vi "GC init.vi"(11 "Serial Port":refnum<visa-resource-name>) -> (0 "error":bool, 3 "Serial Port":refnum<visa-resource-name>)   [LabVIEW 2012]
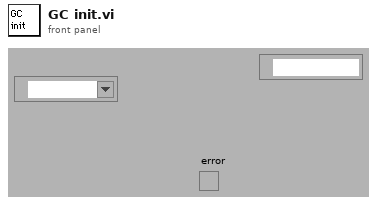
[diagram p1: front panel]
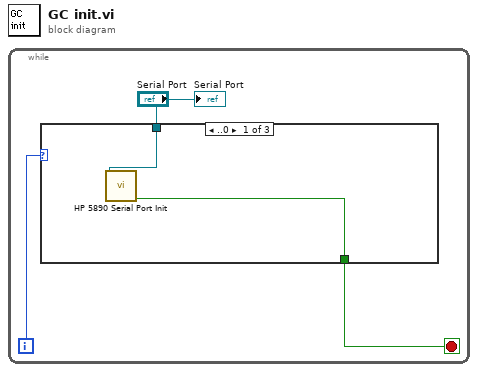
[diagram p0: block diagram]
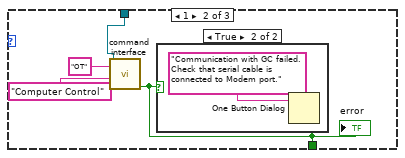
[diagram p2: hidden frame]
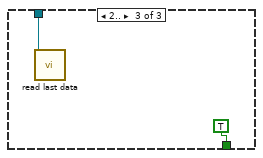
[diagram p4: hidden frame]
diagram:
  n1 = while {
    i -> [w2]
    stop <- w1 stop-if-true
    n2 = case shown="..0" w2 {
      tunnel: "Serial Port" -> [w5 w9 w12]
      tunnel: [w4 w6 TRUE ("timed out")] -> w1
      frame ..0 {
        n3 = call "HP 5890 Serial Port Init.vi"("port number"=w5) -> ("timed out"=w4:bool)  [unwired: 9 in, 1 out]
      }
      frame 1 {
        n4 = call "command interface.vi"("Parameter"="Computer Control", "command"="OT", "Serial Port"=w9) -> ("timed out"=w6:bool)  [unwired: 4 in, 3 out]
        "error" <- w6
        n5 = case shown="True" w6 {
          frame False {
          }
          frame True {
            n6 = One Button Dialog(message="Communication with GC failed. Check that serial cable is connected to Modem port.") -> ()  [unwired: 1 in, 1 out]
          }
        }
      }
      frame 2.. {
        n7 = call "read last data.vi"("Serial Port"=w12) -> ()  [unwired: 9 in, 2 out]
      }
    }
    "Serial Port" <- "Serial Port"
  }
